vi "openbci_channel_count.vi"(8 "error in (no error)":errorcluster, 11 "OBCI dev in":T1={"COM port"="", "n_ch (8)"=enum."8 Channels", "delay_tx"=50}) -> (0 "error out":errorcluster, 3 "OBCI dev out":T1={"COM port"="", "n_ch (8)"=enum."8 Channels", "delay_tx"=50})   [LabVIEW 2013]
doc: "Sends a command for 8 or 16 channels to the OpenBCI board"
uses:
  Control Def/openbci_device.ctl
  Control Def/channel_count.ctl
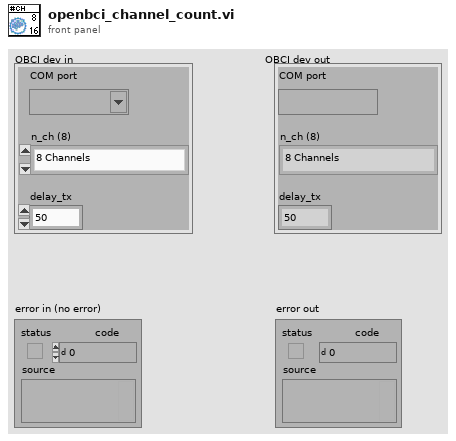
[diagram p1: front panel]
types:
  T1 = typedef "openbci_device.ctl" = cluster{"COM port":refnum<visa-resource-name>, "n_ch (8)":T2, "delay_tx":u32}
  T2 = typedef "channel_count.ctl" = enum16{"8 Channels", "16 Channels"}
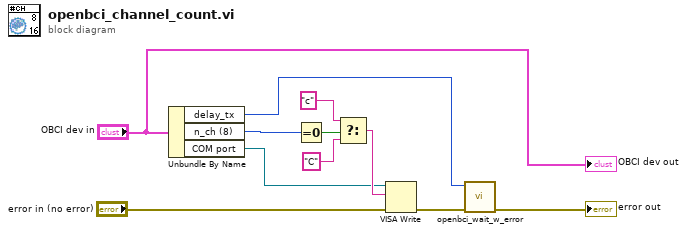
[diagram p0: block diagram]
diagram:
  n1 = Unbundle By Name("OBCI dev in") -> ("delay_tx"=w2:u32, "n_ch (8)"=w5:T2, "COM port"=w6:refnum<visa-resource-name>)
  n2 = Equal To 0?(x=w5) -> (x = 0?=w10:bool)
  n3 = Select(t="c", s=w10, f="C") -> (s? t:f=w8:string)
  n4 = VISA Write(VISA resource name=w6, write buffer=w8, error in (no error)="error in (no error)") -> (error out=w4:errorcluster)  [unwired: 2 out]
  n5 = call "openbci_wait_w_error.vi"("error in (no error)"=w4, "milliseconds to wait"=w2) -> ("error out"=→"error out":errorcluster)  [unwired: 9 in]
  "OBCI dev out" <- "OBCI dev in"
